vi "PtByPtFilter.vi"(0 "parameter cluster":T2={"number of elements"=1, "start value"=0.0, "sinusoidal profile"=[1.0], "gaussian profile"=[1.0]}, 1 "Mode":T1, 5 "demand":dbl=1.0 format="%#_13g", 7 "max speed":dbl=1.0 format="%#_13g", 9 "dt":i64=1, 11 "error in":errorcluster, 12 "reset":bool) -> (6 "filtered signal":dbl format="%#_13g", 15 "error out":errorcluster)   [LabVIEW 2017, in "myPAM.lvlib" / "RealTimeFilter.lvlib"]
uses:
  RealTimeFilter.lvlib
  TypeDefs/Parameters.ctl
  TypeDefs/Modes.ctl
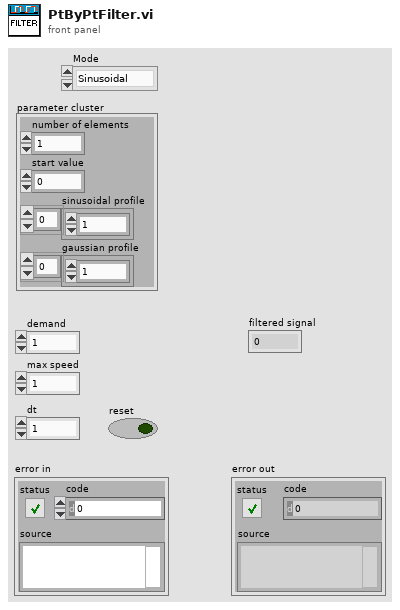
[diagram p1: front panel]
types:
  T1 = typedef "myPAM.lvlib/RealTimeFilter.lvlib/Modes.ctl" = enum16{"Sinusoidal", "Gaussian"}
  T2 = typedef "myPAM.lvlib/RealTimeFilter.lvlib/Parameters.ctl" = cluster{"number of elements":i32, "start value":dbl, "sinusoidal profile":dbl[], "gaussian profile":dbl[]}
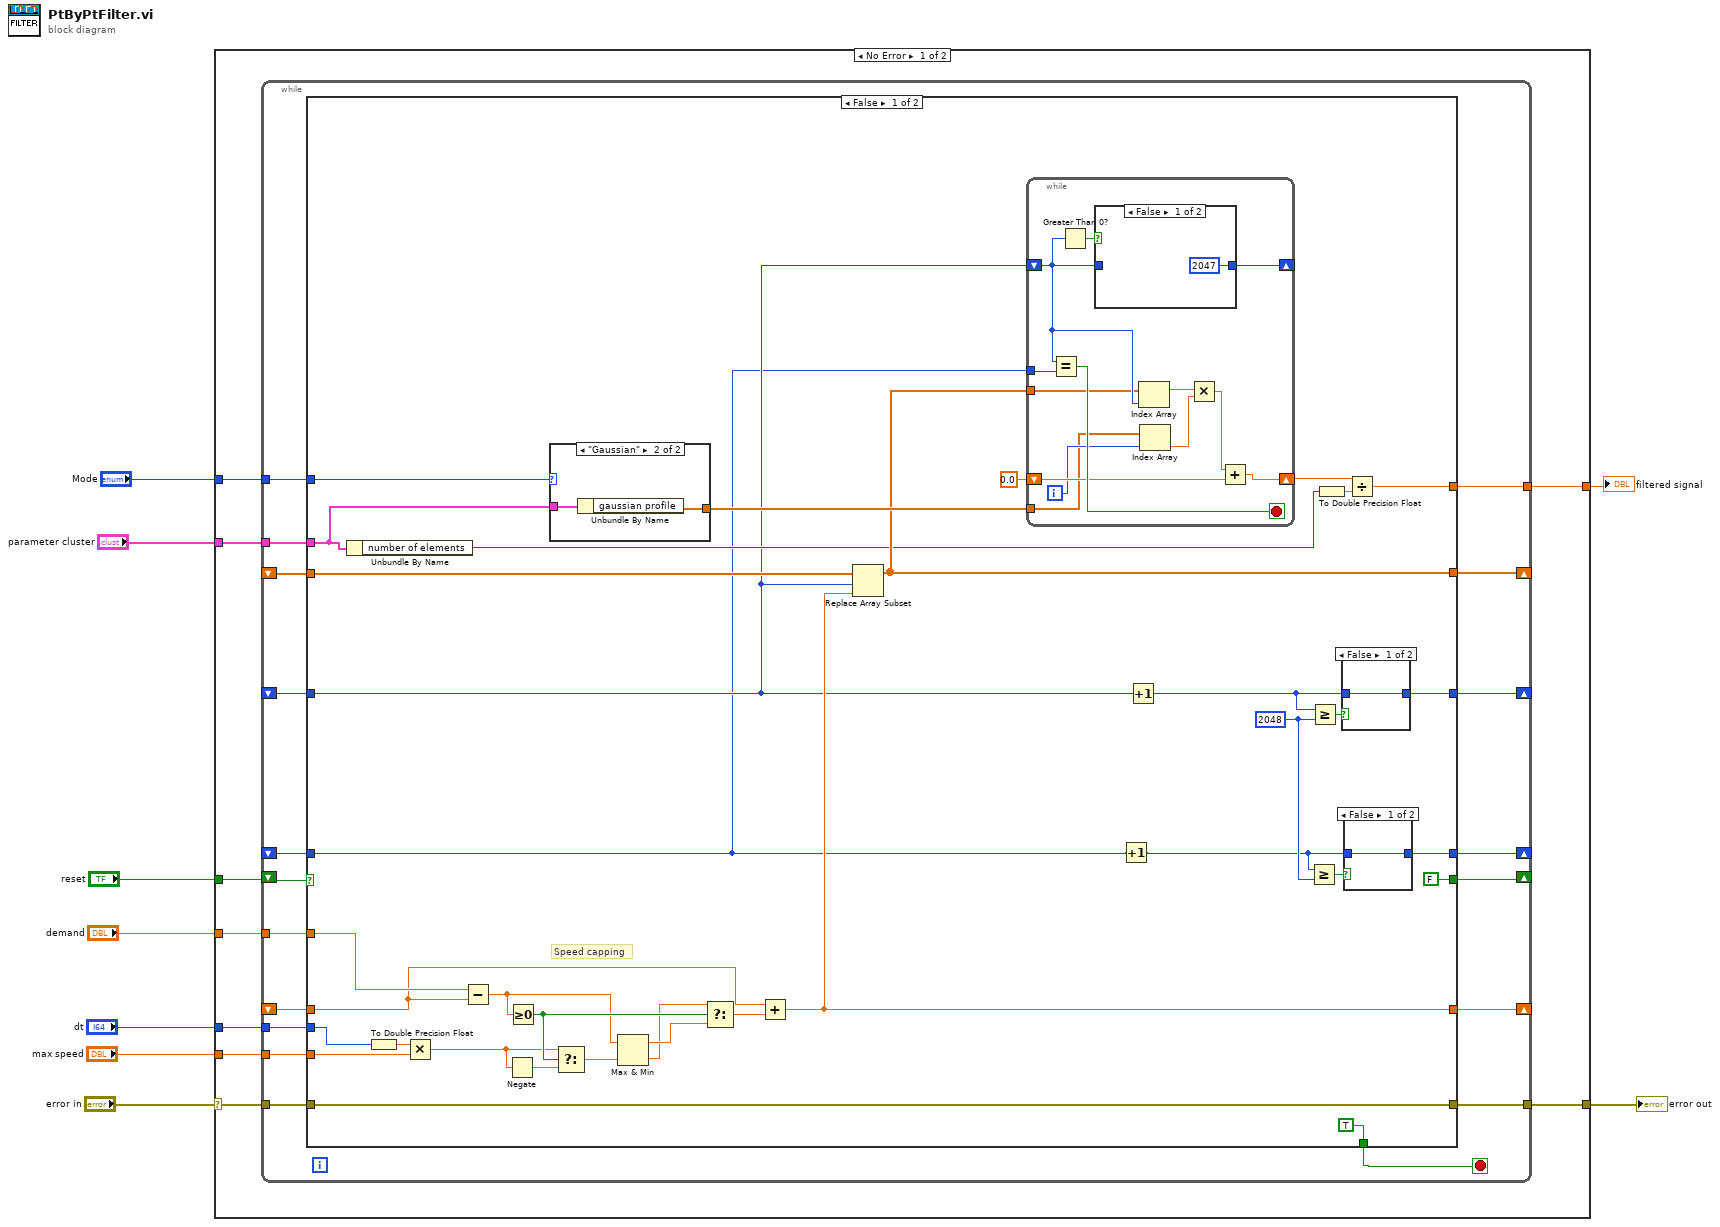
[diagram p0: block diagram]
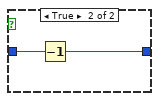
[diagram p2: hidden frame]
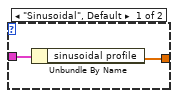
[diagram p3: hidden frame]
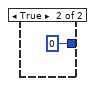
[diagram p4: hidden frame]
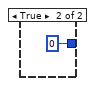
[diagram p5: hidden frame]
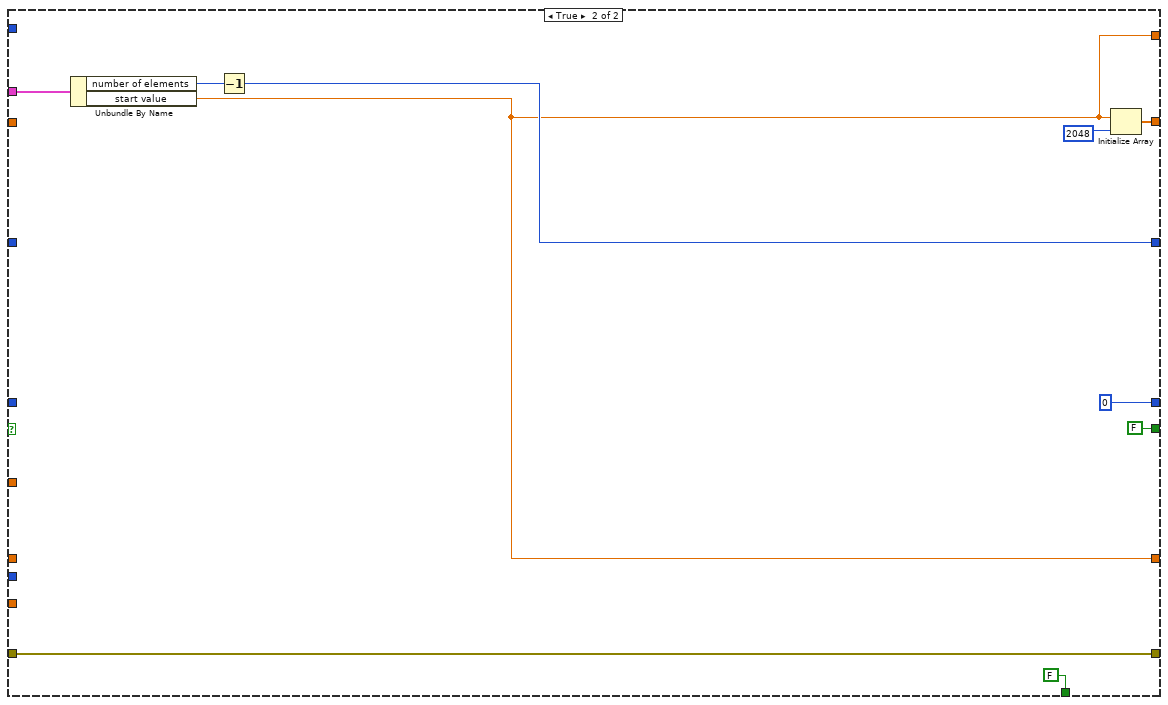
[diagram p6: hidden frame]
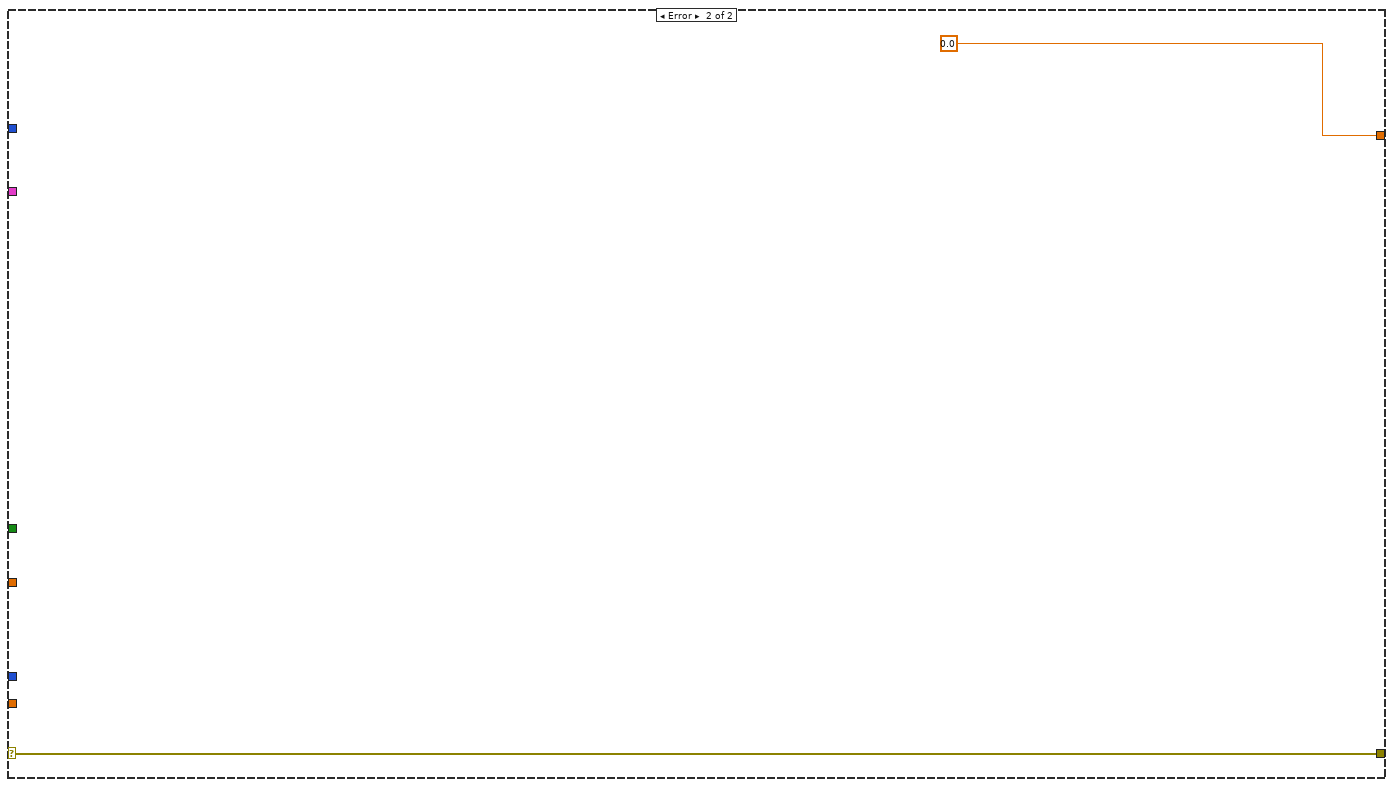
[diagram p7: hidden frame]
diagram:
  n1 = case shown="No Error" "error in" {
    selector: "error in" -> [w14 w109]
    tunnel: "demand" -> [w18 _]
    tunnel: "max speed" -> [w17 _]
    tunnel: "dt" -> [w16 _]
    tunnel: [w15 w109] -> w6
    tunnel: "reset" -> [w13 _]
    tunnel: [w10 0.0 ("filtered signal")] -> w3
    tunnel: "parameter cluster" -> [w12 _]
    tunnel: "Mode" -> [w11 _]
    frame No Error {
      n2 = while {
        tunnel: w18 -> [w35]
        tunnel: w17 -> [w37]
        tunnel: w16 -> [w36]
        shift-right: [w27] -> _
        shift-left: _ -> [w34]
        tunnel: [w25] -> w15
        tunnel: w14 -> [w24]
        shift-right: [w33] -> _
        shift-left: _ -> [w31]
        shift-right: [w32] -> _
        shift-left: _ -> [w30]
        tunnel: w12 -> [w29]
        tunnel: w11 -> [w28]
        shift-right: [w22] -> _
        shift-left: w13 -> [w26]
        shift-right: [w21] -> _
        shift-left: _ -> [w20]
        tunnel: [w19] -> w10
        stop <- w23 stop-if-true
        n3 = case shown="False" w26 {
          tunnel: w37 -> [w67 _]
          tunnel: w36 -> [w66 _]
          tunnel: w35 -> [w62 _]
          tunnel: w34 -> [w61 _]
          tunnel: [w60 w99] -> w33
          tunnel: [w59 0 ("t")] -> w32
          tunnel: w31 -> [w41 _]
          tunnel: w30 -> [w39 _]
          tunnel: w29 -> [w42 w106]
          tunnel: w28 -> [w58 _]
          tunnel: [w53 w98] -> w27
          tunnel: [w51 w105] -> w25
          tunnel: w24 -> [w51 w105]
          tunnel: [TRUE FALSE] -> w23
          tunnel: [FALSE FALSE] -> w22
          tunnel: [w48 w101] -> w21
          tunnel: w20 -> [w47 _]
          tunnel: [w43 w98] -> w19
          frame False {
            w55 = 2048
            # "Speed capping"
            n4 = Unbundle By Name(w42) -> ("number of elements"=w44:i32)
            n5 = To Double Precision Float(number=w66) -> (double precision float=w65:dbl)
            n6 = Multiply(x=w65, y=w67) -> (x*y=w64:dbl)
            n7 = Subtract(x=w62, y=w61) -> (x-y=w68:dbl)
            n8 = Negate(x=w64) -> (-x=w73:dbl)
            n9 = Greater Or Equal To 0?(x=w68) -> (x >= 0?=w71:bool)
            n10 = case shown="\"Gaussian\"" w58 {
              tunnel: [w90 w92] -> w54
              tunnel: w42 -> [w91 w93]
              frame "Sinusoidal", Default {
                n11 = Unbundle By Name(w91) -> ("sinusoidal profile"=w90:dbl[])
              }
              frame "Gaussian" {
                n12 = Unbundle By Name(w93) -> ("gaussian profile"=w92:dbl[])
              }
            }
            n13 = Select(t=w64, s=w71, f=w73) -> (s? t:f=w72:dbl)
            n14 = Max & Min(x=w68, y=w72) -> (max(x,y)=w70:dbl, min(x,y)=w69:dbl)
            n15 = Select(t=w69, s=w71, f=w70) -> (s? t:f=w63:dbl)
            n16 = Add(x=w61, y=w63) -> (x+y=w53:dbl)
            n17 = Replace Array Subset(array=w47, new element=w53, index=w41) -> (w48:dbl[])
            n18 = while {
              shift-right: [w85] -> _
              shift-left: w41 -> [w77]
              tunnel: w39 -> [w84]
              shift-right: [w80] -> w46
              shift-left: 0.0 -> [w82]
              tunnel: w54 -> [w76]
              tunnel: w48 -> [w74]
              i -> [w79]
              stop <- w83 stop-if-true
              n19 = Equal?(x=w77, y=w84) -> (x = y?=w83:bool)
              n20 = Greater Than 0?(x=w77) -> (x > 0?=w86:bool)
              n21 = case shown="False" w86 {
                tunnel: w77 -> [_ w89]
                tunnel: [2047 w88] -> w85
                frame False {
                }
                frame True {
                  n22 = Decrement(x=w89) -> (x-1=w88:i32)
                }
              }
              n23 = Index Array(array=w74, index=w77) -> (element=w78:dbl)
              n24 = Index Array(array=w76, index=w79) -> (element=w75:dbl)
              n25 = Multiply(x=w78, y=w75) -> (x*y=w81:dbl)
              n26 = Add(x=w81, y=w82) -> (x+y=w80:dbl)
            }
            n27 = Increment(x=w39) -> (x+1=w38:i32)
            n28 = Increment(x=w41) -> (x+1=w40:i32)
            n29 = Greater Or Equal?(x=w38, y=w55) -> (x >= y?=w57:bool)
            n30 = Greater Or Equal?(x=w40, y=w55) -> (x >= y?=w56:bool)
            n31 = To Double Precision Float(number=w44) -> (double precision float=w45:dbl)
            n32 = case shown="False" w56 {
              tunnel: w40 -> [w96 _]
              tunnel: [w96 0] -> w60
              frame False {
              }
              frame True {
              }
            }
            n33 = case shown="False" w57 {
              tunnel: [w94 0] -> w59
              tunnel: w38 -> [w94 _]
              frame False {
              }
              frame True {
              }
            }
            n34 = Divide(x=w46, y=w45) -> (x/y=w43:dbl)
          }
          frame True {
            n35 = Unbundle By Name(w106) -> ("number of elements"=w100:i32, "start value"=w98:dbl)
            n36 = Decrement(x=w100) -> (x-1=w99:i32)
            n37 = Initialize Array(w98, 2048) -> (w101:dbl[])
          }
        }
      }
    }
    frame Error {
    }
  }
  "filtered signal" <- w3
  "error out" <- w6
